vi "Launcher.vi"   [LabVIEW 2014, in "Controller.lvclass"]
uses:
  Controller.lvclass
  <vilib>/ActorFramework/Actor/Actor.lvclass
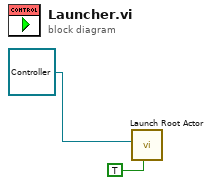
[diagram p0: block diagram]
diagram:
  n1 = call <vilib>:"Launch Root Actor.vi"("Open Actor Core front panel? (F)"=TRUE, "Actor"=refnum<class "Controller.lvclass"> refnum ("Controller.lvclass")) -> ()  [unwired: 8 in, 2 out]
